vi "SampleMaster.vi"() -> ()   [LabVIEW 2012]
doc: "A sample master that can be run on the computer or RIO"
panel:
  out "ms/it":u32(graph)
  out "iteration":i32
  in  "Service call":bool
  in  "Show Web":bool
  in  "Show Node":bool
  out "Answer":string
  in  "LED":bool
  out "LED reply":string
  out "time":string
  out "Status":string
  in  "stop":bool
  # "Instructions:\n1. Run the VI\n2. Verify that you see the correct time.\n3. Press the LED button. You should see the LED reply change.\nIf you are targetting a myRIO, the LED should change as well.\n4. Debug by clicking Show Node and Show Webpage.\n5. See what is being sent back and forth by clicking Show Node and Show Webpage."
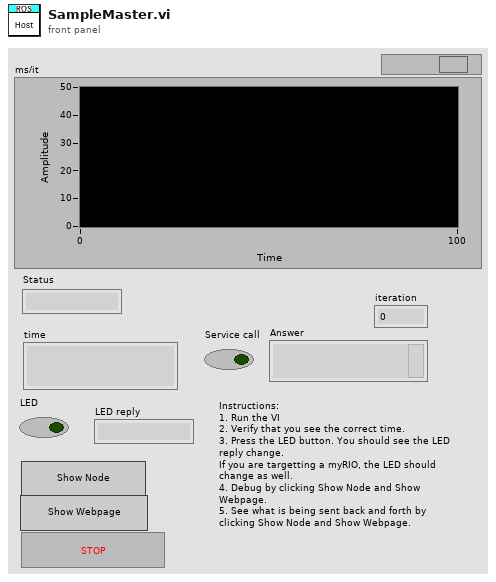
[diagram p1: front panel]
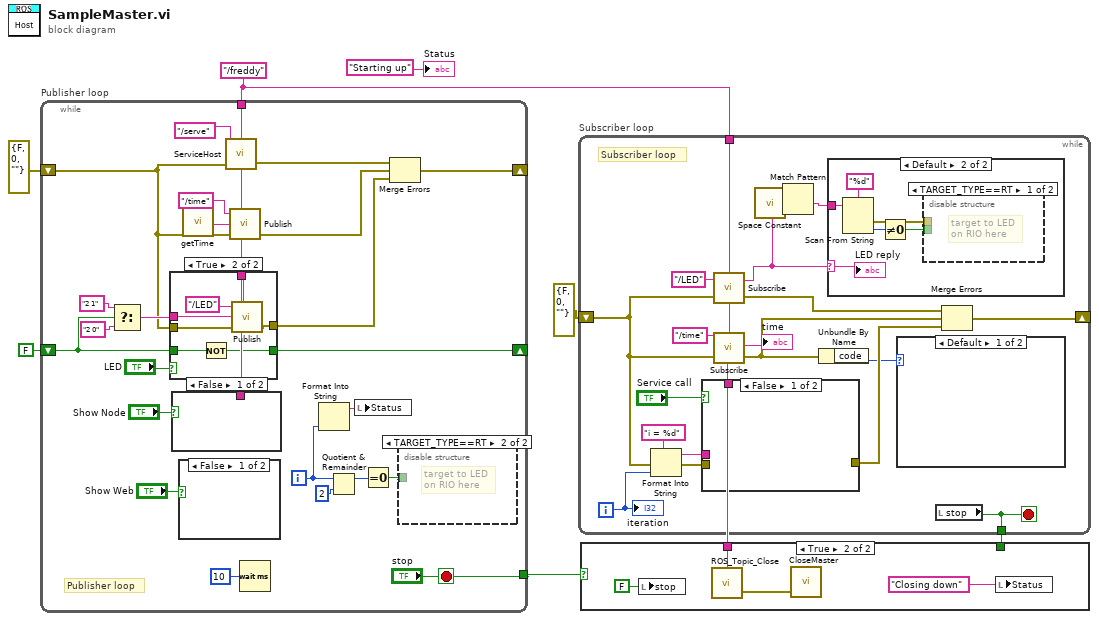
[diagram p0: block diagram]
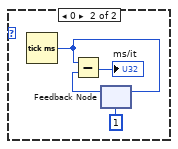
[diagram p2: hidden frame]
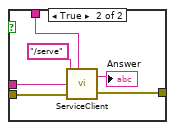
[diagram p5: hidden frame]
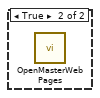
[diagram p8: hidden frame]
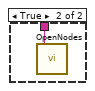
[diagram p10: hidden frame]
diagram:
  w4 = "/freddy" ("Topic")
  n1 = while "Publisher loop" {
    tunnel: ["stop"] -> w5
    tunnel: w4 -> [w19]
    shift-right: [w27] -> _
    shift-left: FALSE -> [w26]
    shift-right: [w12] -> _
    shift-left: errorcluster {"status"=FALSE, "code"=0, "source"=""} ("error out") -> [w10]
    i -> [w15]
    stop <- "stop" stop-if-true
    # "Publisher loop"
    n2 = Select(t="2 1" ("Status"), s=w26, f="2 0" ("Status")) -> (s? t:f=w28:string)
    n3 = case shown="True" "LED" {
      tunnel: w19 -> [_ w37]
      tunnel: w28 -> [_ w36]
      tunnel: [w32 w38] -> w27
      tunnel: w26 -> [w32 w39]
      tunnel: [_ w35] -> w11
      tunnel: w10 -> [_ w33]
      frame False {
      }
      frame True {
        n4 = Not(x=w39) -> (.not. x?=w38:bool)
        n5 = call "Publish.vi"("Topic"="/LED", "node"=w37, "String"=w36, "error in"=w33) -> ("error"=w35:errorcluster)  [unwired: 3 in]
      }
    }
    n6 = case shown="False" "Show Node" {
      tunnel: w19 -> [_ w40]
      frame False {
      }
      frame True {
        n7 = call "OpenNodes.vi"("Node Name"=w40) -> ()  [unwired: 1 in]
      }
    }
    n8 = case shown="False" "Show Web" {
      frame False {
      }
      frame True {
        n9 = call "OpenMasterWebPages.vi"() -> ()  [unwired: 4 in]
      }
    }
    n10 = call "getTime.vi"() -> ("Current Time"=w21:string)  [unwired: 1 in]
    n11 = call "ServiceHost.vi"("error in"=w10, "Topic"="/serve", "node"=w19) -> ("error out"=w14:errorcluster)  [unwired: 1 out]
    n12 = call "Publish.vi"("Topic"="/time", "node"=w19, "String"=w21, "error in"=w10) -> ("error"=w13:errorcluster)  [unwired: 3 in]
    n13 = Wait (ms)(milliseconds to wait=u32 10) -> ()  [unwired: 1 out]
    n14 = Format Into String(w15) -> (resulting string=w31:string)  [unwired: 3 in, 1 out]
    n15 = Quotient & Remainder(x=w15, y=2) -> (x-y*floor(x/y)=w17:i32)  [unwired: 1 out]
    n16 = local write "Status"(w31) -> ()
    n17 = Equal To 0?(x=w17) -> (x = 0?=w16:bool)
    n18 = Merge Errors(w14, w13, w11) -> (w12:errorcluster)
    n19 = disable-structure shown="TARGET_TYPE==RT" {
      disable-tunnel: w16 -> [_ _]
      frame condition #0 (active) {
      }
      frame condition #1 {
        # "target to LED\non RIO here"
      }
    }
  }
  n20 = while "Subscriber loop" {
    tunnel: w4 -> [w50]
    shift-right: [w46] -> _
    shift-left: errorcluster {"status"=FALSE, "code"=0, "source"=""} ("error out") -> [w45]
    tunnel: [w47] -> w1
    i -> [w54]
    stop <- w47 stop-if-true
    # "Subscriber loop"
    n21 = Format Into String(format string="i = %d" ("Msg in"), w54) -> (resulting string=w53:string)  [unwired: 2 in, 1 out]
    n22 = case shown="False" "Service call" {
      tunnel: [_ w73] -> w43
      tunnel: w53 -> [_ w72]
      tunnel: w50 -> [_ w71]
      tunnel: w45 -> [_ w70]
      frame False {
      }
      frame True {
        n23 = call "ServiceClient.vi"("Topic"="/serve", "node"=w71, "Msg in"=w72, "error in"=w70) -> ("Reply"=→"Answer":string, "error out"=w73:errorcluster)  [unwired: 1 in]
      }
    }
    n24 = call "Subscribe.vi"("error in"=w45, "Topic"="/LED", "node"=w50) -> ("error out"=w44:errorcluster, "Reply"=w49:string)
    n25 = call "Subscribe.vi"("error in"=w45, "Topic"="/time", "node"=w50) -> ("error out"=w41:errorcluster, "Reply"=→"time":string)
    n26 = call <vilib>:"Space Constant.vi"() -> ("String"=w56:string)
    n27 = Match Pattern(string=w49, regular expression=w56) -> (after substring=w55:string)  [unwired: 1 in, 3 out]
    n28 = Unbundle By Name(w41) -> ("code"=w42:i32)
    n29 = case shown="Default" w49 {
      selector: w49 -> [_ w63]
      tunnel: w55 -> [_ w68]
      frame "" {
      }
      frame Default {
        n30 = Scan From String(format string="%d", input string=w68) -> (error out=w64:errorcluster, output 1=w66:i32)  [unwired: 3 in, 2 out]
        n31 = Not Equal To 0?(x=w66) -> (x != 0?=w65:bool)
        n32 = disable-structure shown="TARGET_TYPE==RT" {
          disable-tunnel: w65 -> [_ _]
          disable-tunnel: w64 -> [_ _]
          frame condition #0 {
            # "target to LED\non RIO here"
          }
          frame condition #1 (active) {
          }
        }
        "LED reply" <- w63
      }
    }
    n33 = case shown="Default" w42 {
      frame Default {
      }
      frame 0 {
        n34 = Tick Count (ms)() -> (millisecond timer value=w61:u32)
        n35 = feedback-in #1(w61) -> ()
        n36 = feedback #1(u32 1 ("milliseconds to wait")) -> (w60:u32)
        n37 = Subtract(x=w61, y=w60) -> (x-y=→"ms/it":u32)
      }
    }
    n38 = local read "stop"() -> (w47:bool)
    n39 = Merge Errors(w44, w41, w43) -> (w46:errorcluster)
    "iteration" <- w54
  }
  n40 = case shown="True" w5 {
    tunnel: w4 -> [_ w77]
    tunnel: w1 -> [_ _]
    frame False {
    }
    frame True {
      n41 = local write "stop"(FALSE ("stop")) -> ()
      n42 = call "ROS_Topic_Close.vi"("node"=w77) -> ("error out"=w76:errorcluster)  [unwired: 3 in]
      n43 = call "CloseMaster.vi"("error in (no error)"=w76) -> ()  [unwired: 2 in, 1 out]
      n44 = local write "Status"("Closing down" ("Status")) -> ()
    }
  }
  "Status" <- "Starting up" ("Status")
